vi "Destroy.vi"(8 "error in (no error)":errorcluster, 11 "File Sink in":refnum<class "File Sink.lvclass">) -> (0 "error out":errorcluster, 3 "Log File Path":path)   [LabVIEW 2020, in "LV Log.lvlib" / "File Sink.lvclass"]
uses:
  File Sink.lvclass
  File Sink.lvclass/File Sink.ctl
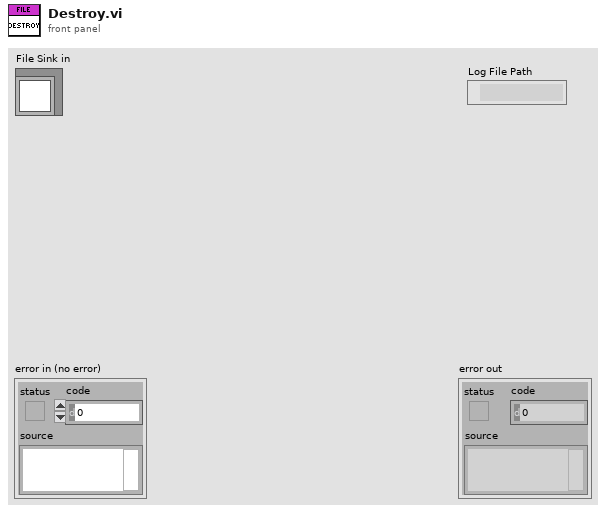
[diagram p1: front panel]
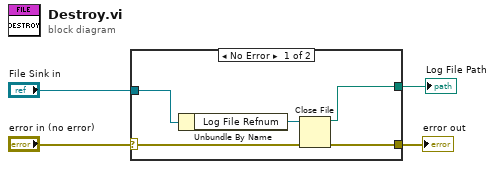
[diagram p0: block diagram]
diagram:
  n1 = case shown="No Error" "error in (no error)" {
    selector: "error in (no error)" -> [w8 w10]
    tunnel: [w7 w10] -> w3
    tunnel: "File Sink in" -> [w6 _]
    tunnel: [w5 _] -> w1
    frame No Error {
      n2 = Unbundle By Name(w6) -> ("Log File Refnum"=w9:refnum<file>)
      n3 = Close File(refnum=w9, error in=w8) -> (path=w5:path, error out=w7:errorcluster)
    }
    frame Error {
    }
  }
  "error out" <- w3
  "Log File Path" <- w1
